vi "UpdateMCListboxFromControls.vi"(6 "IncludeSymbols?":bool=TRUE, 8 "error in (no error)":errorcluster, 10 "Controls":T1[](array[typedef]), 11 "MulticolumnListbox in":refnum<vi>) -> (0 "error out":errorcluster)   [LabVIEW 2020, in "ContextHelpEditor.lvlib"]
uses:
  ContextHelpEditor.lvlib
  ControlRef--cluster.ctl
  <vilib>/picture/picture.llb/imagedata.ctl
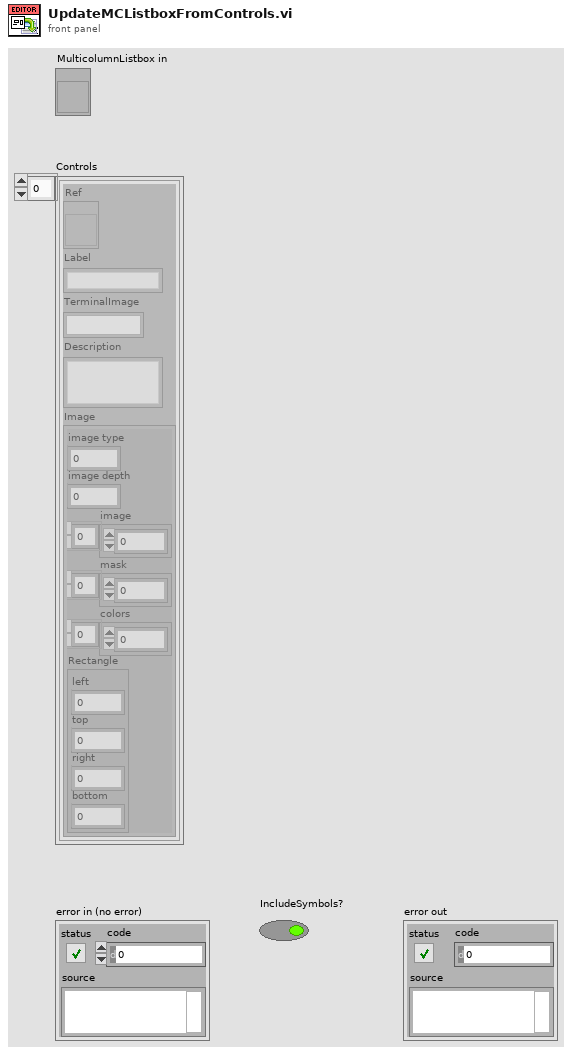
[diagram p1: front panel]
types:
  T1 = typedef "ContextHelpEditor.lvlib/ControlRef--cluster.ctl" = cluster{"Ref":refnum<vi>, "Label":string, "TerminalImage":picture, "Description":string, "Image":T2}
  T2 = typedef "imagedata.ctl" = cluster{"image type":i32, "image depth":i32, "image":u8[], "mask":u8[], "colors":u32[], "Rectangle":cluster{"left":i16, "top":i16, "right":i16, "bottom":i16}}
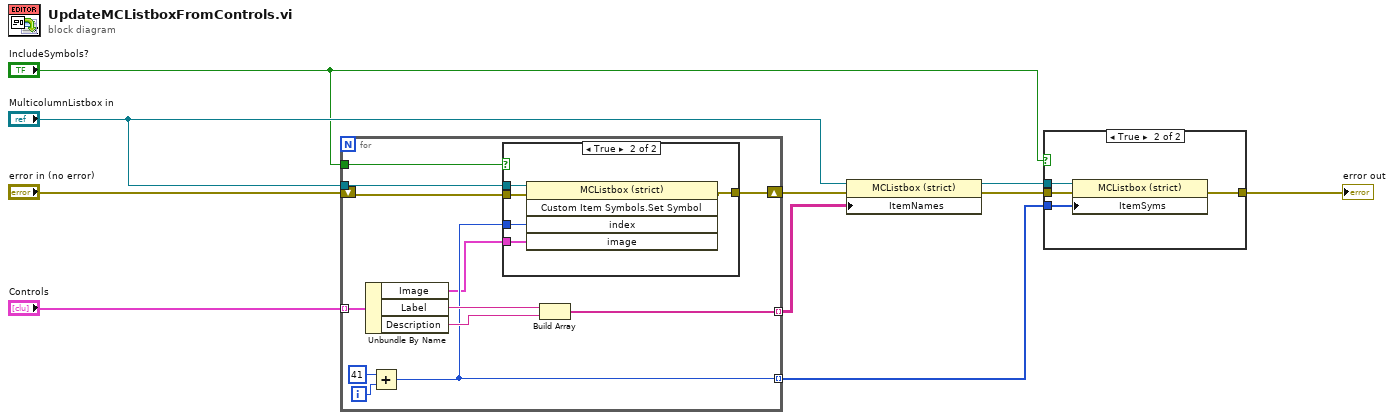
[diagram p0: block diagram]
diagram:
  n1 = for {
    tunnel: "Controls" -> [w22] mode=indexing
    tunnel: [w19] -> w7 mode=indexing
    tunnel: [w16] -> w2 mode=indexing
    tunnel: "MulticolumnListbox in" -> [w12]
    shift-right: [w14] -> w9
    shift-left: "error in (no error)" -> [w13]
    tunnel: "IncludeSymbols?" -> [w11]
    i -> [w18]
    n2 = Unbundle By Name(w22) -> ("Image"=w15:T2, "Label"=w21:string, "Description"=w20:string)
    n3 = Add(x=41, y=w18) -> (x+y=w16:i32)
    n4 = case shown="True" w11 {
      tunnel: w16 -> [_ w28]
      tunnel: w15 -> [_ w27]
      tunnel: [w23 w26] -> w14
      tunnel: w13 -> [w23 w25]
      tunnel: w12 -> [_ w24]
      frame False {
      }
      frame True {
        n5 = invoke class="MCListbox (strict)" method="Custom Item Symbols.Set Symbol"(reference=w24, error in=w25, "index"=w28, "image"=w27) -> (error out=w26:errorcluster)  [unwired: 1 in, 4 out]
      }
    }
    n6 = Build Array(w21, w20) -> (w19:string[])
  }
  n7 = property class="MCListbox (strict)"(reference="MulticolumnListbox in", error in=w9, "ItemNames"=w7) -> (reference out=w5:refnum<vi>, error out=w4:errorcluster)
  n8 = case shown="True" "IncludeSymbols?" {
    tunnel: w5 -> [_ w33]
    tunnel: w4 -> [w29 w32]
    tunnel: [w29 w31] -> w3
    tunnel: w2 -> [_ w30]
    frame False {
    }
    frame True {
      n9 = property class="MCListbox (strict)"(reference=w33, error in=w32, "ItemSyms"=w30) -> (error out=w31:errorcluster)  [unwired: 1 out]
    }
  }
  "error out" <- w3
